vi "General PID with Fault Protection.vi"() -> ()   [LabVIEW 2023]
doc: "This example demonstrates how to simulate a general PID controller in the presence of a faulty measurement, where it will give NaN as measurement. It shows how to add LabVIEW code to avoid the NaN in the PID controller, which will \"lockdown\" the internal state of the controller."
uses:
  <vilib>/addons/control/pid/pid.llb/PID (DBL).vi
  <vilib>/addons/control/pid/NI_PID_pid.lvlib
panel:
  out "Output":dbl(graph)
  in  "SP:":dbl(slide)=54.966887417218544 min=0.0 max=0.0 scale=0.0..100.0
  out "MV:":dbl(slide)=100.0 scale=-100.0..100.0
  out "PV:":dbl(slide)=33.01408837398299 scale=0.0..100.0
  in  "Percentage of\nfailing measurements":dbl=15.0 min=0.0 max=100.0
  out "Measurement\nFault (PVF)":bool
  in  "PID gains":T1={"proportional gain (Kc)"=20.0, "integral time (Ti, min)"=0.008, "derivative time (Td, min)"=0.001} {"derivative time (Td, min)" format="%.3f"; "integral time (Ti, min)" format="%.3f"; "proportional gain (Kc)" format="%.3f"}
  in  "Sampling Time dt (s)":dbl=0.05 min=0.001 step=0.01 format="%#.3p"
  in  "Stop":bool
  out "Input and setpoint":cluster{dbl, "SP:":dbl}(graph)
  # "Overview: This example demonstrates how to simulate a general PID controller in the presence of a faulty measurement, where it will give NaN as measurement. It shows how to add LabVIEW code to avoid the NaN in the PID controller, which will  \"lock down\" the internal state of the controller.\nInstructions:\n1. Run the VI.\n2. Verify that when a Measurement Fault (PVF) happen, the code will avoid the NaN to get into the controller and it would use the previous measurement to avoid this issue.\n3. Increase the Percentage of failing measurements and see that the controller still works, although not as good as with a lower rate.\n4. Click Stop to stop the VI."
  # "%"
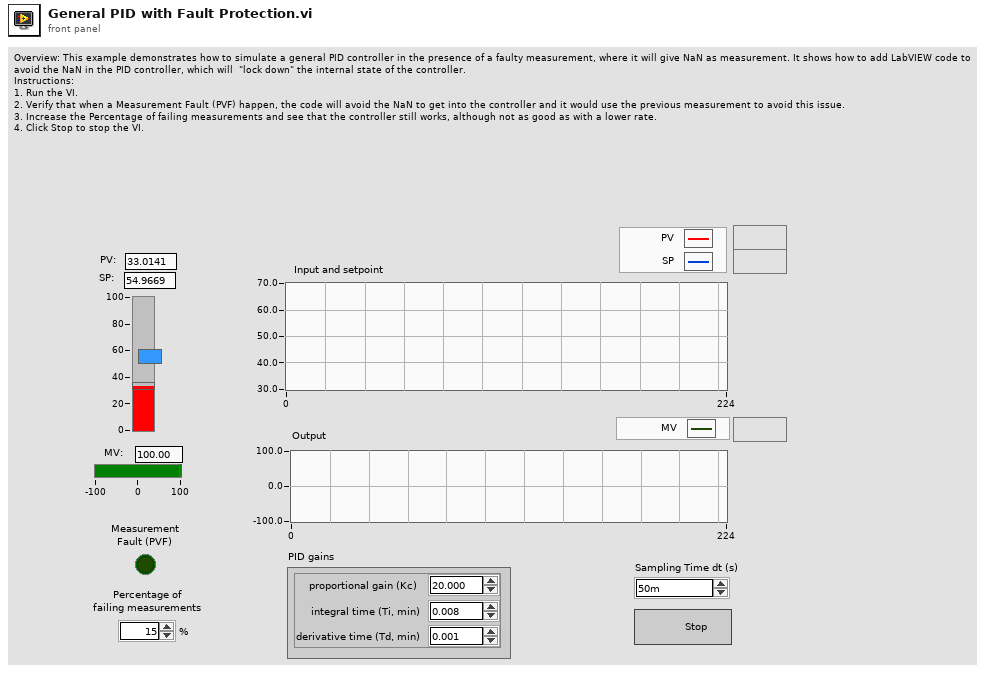
[diagram p1: front panel]
types:
  T1 = cluster{"proportional gain (Kc)":dbl, "integral time (Ti, min)":dbl, "derivative time (Td, min)":dbl}
  T2 = cluster{"static gain":dbl, "lag (min)":dbl, "dead cycles":dbl, "load %":dbl, "deadband":dbl, "noise level %":dbl, "initial PV":dbl, "initial PV 2":dbl}
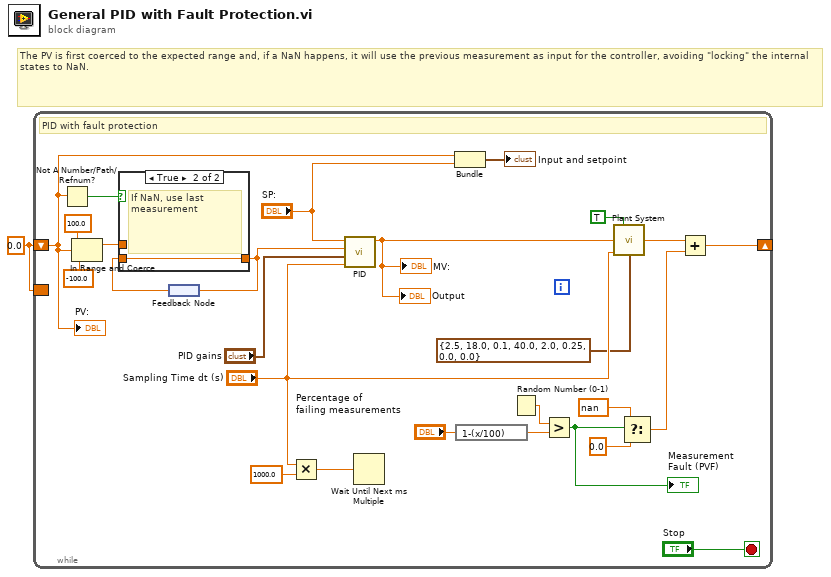
[diagram p0: block diagram]
diagram:
  w1 = 0.0
  # "The PV is first coerced to the expected range and, if a NaN happens, it will use the previous measurement as input for the controller, avoiding \"locking\" the internal states to NaN."
  n1 = while {
    shift-left: w1 -> [w3]
    shift-right: [w16] -> _
    border: w1 -> [_]
    stop <- "Stop" stop-if-true
    # "PID with fault protection"
    n2 = Not A Number/Path/Refnum?(number/path/refnum=w3) -> (NaN/Path/Refnum?=w24:bool)
    n3 = In Range and Coerce(upper limit=100.0, x=w3, lower limit=-100.0) -> (coerced(x)=w10:dbl)  [unwired: 1 out]
    n4 = feedback #1() -> (w23:dbl)
    n5 = case shown="True" w24 {
      tunnel: w10 -> [w28 _]
      tunnel: [w28 w29] -> w4
      tunnel: w23 -> [_ w29]
      frame False {
      }
      frame True {
        # "If NaN, use last measurement"
      }
    }
    n6 = feedback-in #1(w4) -> ()
    n7 = Multiply(x="Sampling Time dt (s)", y=1000.0) -> (x*y=w2:dbl)
    n8 = call-poly <vilib>:"PID.vi"("dt (s)"="Sampling Time dt (s)", "PID gains"="PID gains", "process variable"=w4, "setpoint"="SP:") -> ("output"=w6:dbl)  [unwired: 6 in, 1 out]
    "MV:" <- w6
    "Output" <- w6
    n9 = Wait Until Next ms Multiple(millisecond multiple=w2) -> ()  [unwired: 1 out]
    n10 = Bundle(w3, "SP:"="SP:") -> (→"Input and setpoint":cluster{dbl, "SP:":dbl})  [unwired: 1 in]
    n11 = expression code="1-(x/100)"("Percentage of\nfailing measurements") -> (w14:dbl)
    n12 = Random Number (0-1)() -> (number: 0 to 1=w22:dbl)
    n13 = Greater?(x=w22, y=w14) -> (0:w21:bool)
    "Measurement\nFault (PVF)" <- w21
    n14 = call "Plant System.vi"("Integrator ?"=TRUE, "Plant Input"=w6, "dt (s)"="Sampling Time dt (s)", "process parameters"=T2 {"static gain"=2.5, "lag (min)"=18.0, "dead cycles"=0.1, "load %"=40.0, "deadband"=2.0, "noise level %"=0.25, "initial PV"=0.0, "initial PV 2"=0.0}) -> ("Plant Output"=w17:dbl)  [unwired: 11 in]
    n15 = Select(t=nan, s=w21, f=0.0) -> (s? t:f=w18:dbl)
    n16 = Add(x=w17, y=w18) -> (x+y=w16:dbl)
    "PV:" <- w3
  }
